vi "MysqlTest2 (2).vi"() -> ()   [LabVIEW 2018]
uses:
  Subvi/TheConnWithOmron/Panel_IO.ctl
  Subvi/TheConnWithOmron/Panel_IO2.ctl
  <vilib>/addons/database/Connection.llb/DB Tools Open Connec (String).vi
  <vilib>/addons/database/NI_Database_API.lvlib
panel:
  out "连接的字符串":string
  in  "终止":bool
  in  "左侧菜单选项卡":T1
  in  "重新连接":bool
  out "连接信号":bool
  in  "用户变更":bool
  in  "请选择用户:":enum16{"", "Operator", "Administrator"}(ring)
  in  "请输入密码:":string
  in  "确认变更":bool
  out "当前用户:":enum16{"Null", "Operator", "Administrator"}(ring)
  in  "用户登出":bool
  out "伺服参数监控":string[](array[string])
  in  "4":bool
  in  "3":bool
  in  "2":bool
  in  "1":bool
  in  "主界面选项卡":enum32{"IO监控", "参数设置", "手动操作", "数据管理", "调试界面"}(tab)
  in  "IO监控滚动条":i32(c297)
  out "Input":T2
  out "Output":T3
  in  "查询":bool
  in  "终结时间":timestamp
  in  "起始时间":timestamp
  in  "关键字查询":string
  in  "刷新":bool
  out "当前页数":i16
  out "总页数":i16
  in  "下一页":bool
  in  "上一页":bool
  out "数据查询":string[][](table)
  out "data":string[][](table)
  out "error out":errorcluster caption="错误输出"
  out "ExcelOutputData":string[](array[string])
  out "ExcelInputData":string[](array[string])
  out "InputData":string[][](array[string])
  out "引用输出":refnum<k24>
  out "OuputData":string[][](array[string])
  out "MachineCondition":string[][](array[string])
  # "mm"
  # "X1Pos:"
  # "mm"
  # "X2Pos:"
  # "mm"
  # "X3Pos:"
  # "mm"
  # "X4Pos:"
  # "mm"
  # "X5Pos:"
  # "mm"
  # "X6Pos:"
  # "mm"
  # "X7Pos:"
  # "mm/s"
  # "X1Vel:"
  # "mm/s"
  # "X2Vel:"
  # "mm/s"
  # "X3Vel:"
  # "mm/s"
  # "X4Vel:"
  # "mm/s"
  # "X5Vel:"
  # "mm/s"
  # "X6Vel:"
  # "mm/s"
  # "X7Vel:"
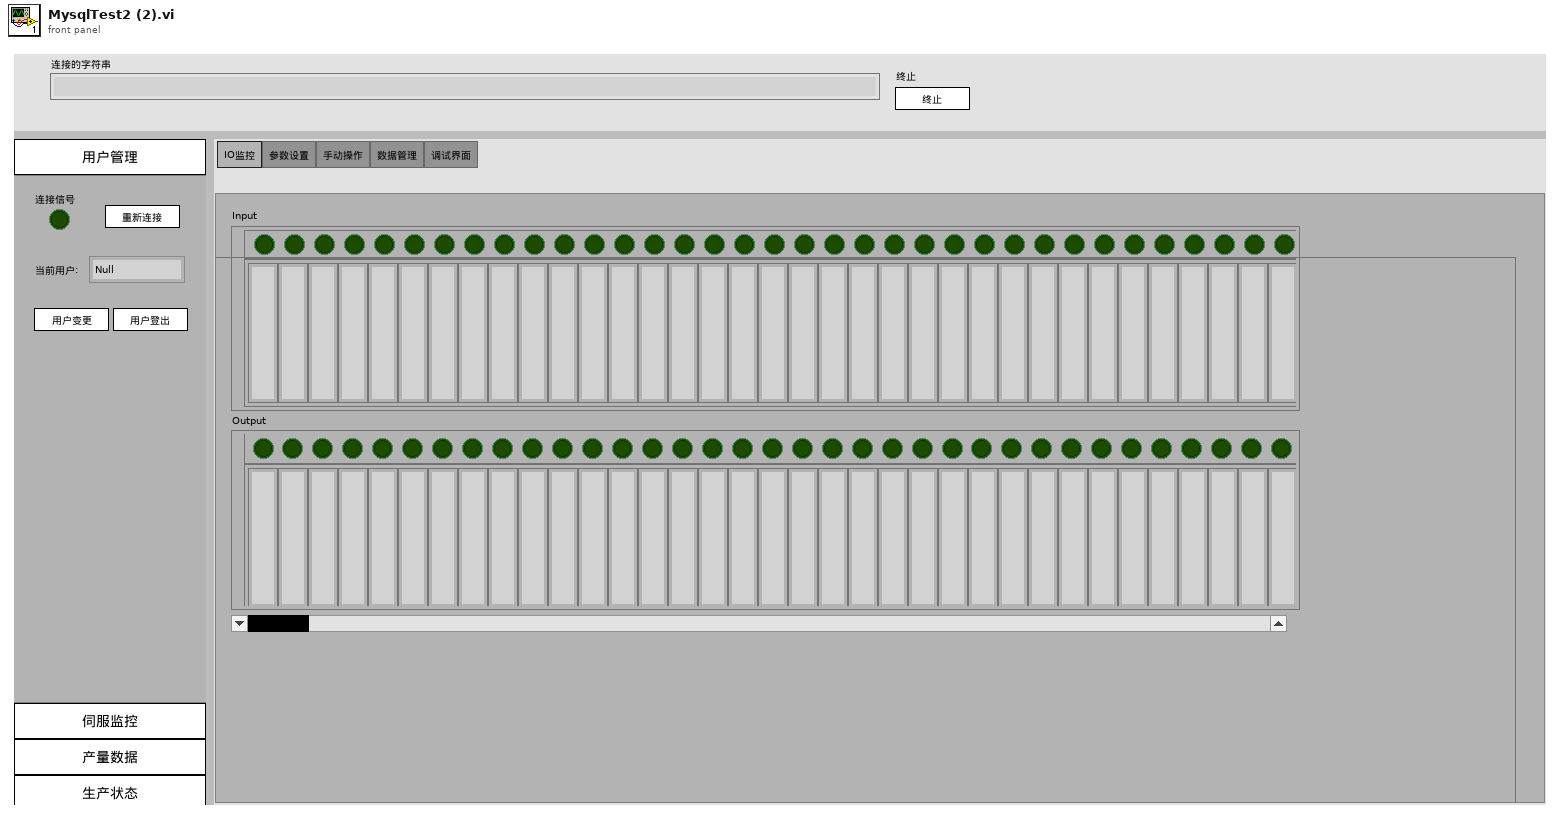
[diagram p1: front panel]
types:
  T1 = typedef "左侧菜单栏选项卡.ctl" = enum32{"用户管理", "伺服监控", "产量数据", "状态监控"}
  T2 = typedef "Panel_IO2.ctl" = cluster{"InputContent":cluster{"InputContent[0]":bool, "InputContent[1]":bool, "InputContent[2]":bool, "InputContent[3]":bool, "InputContent[4]":bool, "InputContent[5]":bool, "InputContent[6]":bool, "InputContent[7]":bool, "InputContent[8]":bool, "InputContent[9]":bool, "InputContent[10]":bool, "InputContent[11]":bool, "InputContent[12]":bool, "InputContent[13]":bool, "InputContent[14]":bool, "InputContent[15]":bool, "InputContent[16]":bool, "InputContent[17]":bool, "InputContent[18]":bool, "InputContent[19]":bool, "InputContent[20]":bool, "InputContent[21]":bool, "InputContent[22]":bool, "InputContent[23]":bool, "InputContent[24]":bool, "InputContent[25]":bool, "InputContent[26]":bool, "InputContent[27]":bool, "InputContent[28]":bool, "InputContent[29]":bool, "InputContent[30]":bool, "InputContent[31]":bool, "InputContent[32]":bool, "InputContent[33]":bool, "InputContent[34]":bool, "InputContent[35]":bool, "InputContent[36]":bool, "InputContent[37]":bool, "InputContent[38]":bool, "InputContent[39]":bool, "InputContent[40]":bool, "InputContent[41]":bool, "InputContent[42]":bool, "InputContent[43]":bool, "InputContent[44]":bool, "InputContent[45]":bool, "InputContent[46]":bool, "InputContent[47]":bool, "InputContent[48]":bool, "InputContent[49]":bool, "InputContent[50]":bool, "InputContent[51]":bool, "InputContent[52]":bool, "InputContent[53]":bool, "InputContent[54]":bool, "InputContent[55]":bool, "InputContent[56]":bool, "InputContent[57]":bool, "InputContent[58]":bool, "InputContent[59]":bool, "InputContent[60]":bool, "InputContent[61]":bool, "InputContent[62]":bool, "InputContent[63]":bool, "InputContent[64]":bool, "InputContent[65]":bool, "InputContent[66]":bool, "InputContent[67]":bool, "InputContent[68]":bool, "InputContent[69]":bool, "InputContent[70]":bool, "InputContent[71]":bool}, "ExcelInputData":cluster{"ExcelInputData[0]":string, "ExcelInputData[1]":string, "ExcelInputData[2]":string, "ExcelInputData[3]":string, "ExcelInputData[4]":string, "ExcelInputData[5]":string, "ExcelInputData[6]":string, "ExcelInputData[7]":string, "ExcelInputData[8]":string, "ExcelInputData[9]":string, "ExcelInputData[10]":string, "ExcelInputData[11]":string, "ExcelInputData[12]":string, "ExcelInputData[13]":string, "ExcelInputData[14]":string, "ExcelInputData[15]":string, "ExcelInputData[16]":string, "ExcelInputData[17]":string, "ExcelInputData[18]":string, "ExcelInputData[19]":string, "ExcelInputData[20]":string, "ExcelInputData[21]":string, "ExcelInputData[22]":string, "ExcelInputData[23]":string, "ExcelInputData[24]":string, "ExcelInputData[25]":string, "ExcelInputData[26]":string, "ExcelInputData[27]":string, "ExcelInputData[28]":string, "ExcelInputData[29]":string, "ExcelInputData[30]":string, "ExcelInputData[31]":string, "ExcelInputData[32]":string, "ExcelInputData[33]":string, "ExcelInputData[34]":string, "ExcelInputData[35]":string, "ExcelInputData[36]":string, "ExcelInputData[37]":string, "ExcelInputData[38]":string, "ExcelInputData[39]":string, "ExcelInputData[40]":string, "ExcelInputData[41]":string, "ExcelInputData[42]":string, "ExcelInputData[43]":string, "ExcelInputData[44]":string, "ExcelInputData[45]":string, "ExcelInputData[46]":string, "ExcelInputData[47]":string, "ExcelInputData[48]":string, "ExcelInputData[49]":string, "ExcelInputData[50]":string, "ExcelInputData[51]":string, "ExcelInputData[52]":string, "ExcelInputData[53]":string, "ExcelInputData[54]":string, "ExcelInputData[55]":string, "ExcelInputData[56]":string, "ExcelInputData[57]":string, "ExcelInputData[58]":string, "ExcelInputData[59]":string, "ExcelInputData[60]":string, "ExcelInputData[61]":string, "ExcelInputData[62]":string, "ExcelInputData[63]":string, "ExcelInputData[64]":string, "ExcelInputData[65]":string, "ExcelInputData[66]":string, "ExcelInputData[67]":string, "ExcelInputData[68]":string, "ExcelInputData[69]":string, "ExcelInputData[70]":string, "ExcelInputData[71]":string}}
  T3 = typedef "Panel_IO.ctl" = cluster{"OutputContent":cluster{"OutputContent[0]":bool, "OutputContent[1]":bool, "OutputContent[2]":bool, "OutputContent[3]":bool, "OutputContent[4]":bool, "OutputContent[5]":bool, "OutputContent[6]":bool, "OutputContent[7]":bool, "OutputContent[8]":bool, "OutputContent[9]":bool, "OutputContent[10]":bool, "OutputContent[11]":bool, "OutputContent[12]":bool, "OutputContent[13]":bool, "OutputContent[14]":bool, "OutputContent[15]":bool, "OutputContent[16]":bool, "OutputContent[17]":bool, "OutputContent[18]":bool, "OutputContent[19]":bool, "OutputContent[20]":bool, "OutputContent[21]":bool, "OutputContent[22]":bool, "OutputContent[23]":bool, "OutputContent[24]":bool, "OutputContent[25]":bool, "OutputContent[26]":bool, "OutputContent[27]":bool, "OutputContent[28]":bool, "OutputContent[29]":bool, "OutputContent[30]":bool, "OutputContent[31]":bool, "OutputContent[32]":bool, "OutputContent[33]":bool, "OutputContent[34]":bool, "OutputContent[35]":bool, "OutputContent[36]":bool, "OutputContent[37]":bool, "OutputContent[38]":bool, "OutputContent[39]":bool, "OutputContent[40]":bool, "OutputContent[41]":bool, "OutputContent[42]":bool, "OutputContent[43]":bool, "OutputContent[44]":bool, "OutputContent[45]":bool, "OutputContent[46]":bool, "OutputContent[47]":bool}, "ExcelOutputData":cluster{"ExcelOutputData[0]":string, "ExcelOutputData[1]":string, "ExcelOutputData[2]":string, "ExcelOutputData[3]":string, "ExcelOutputData[4]":string, "ExcelOutputData[5]":string, "ExcelOutputData[6]":string, "ExcelOutputData[7]":string, "ExcelOutputData[8]":string, "ExcelOutputData[9]":string, "ExcelOutputData[10]":string, "ExcelOutputData[11]":string, "ExcelOutputData[12]":string, "ExcelOutputData[13]":string, "ExcelOutputData[14]":string, "ExcelOutputData[15]":string, "ExcelOutputData[16]":string, "ExcelOutputData[17]":string, "ExcelOutputData[18]":string, "ExcelOutputData[19]":string, "ExcelOutputData[20]":string, "ExcelOutputData[21]":string, "ExcelOutputData[22]":string, "ExcelOutputData[23]":string, "ExcelOutputData[24]":string, "ExcelOutputData[25]":string, "ExcelOutputData[26]":string, "ExcelOutputData[27]":string, "ExcelOutputData[28]":string, "ExcelOutputData[29]":string, "ExcelOutputData[30]":string, "ExcelOutputData[31]":string, "ExcelOutputData[32]":string, "ExcelOutputData[33]":string, "ExcelOutputData[34]":string, "ExcelOutputData[35]":string, "ExcelOutputData[36]":string, "ExcelOutputData[37]":string, "ExcelOutputData[38]":string, "ExcelOutputData[39]":string, "ExcelOutputData[40]":string, "ExcelOutputData[41]":string, "ExcelOutputData[42]":string, "ExcelOutputData[43]":string, "ExcelOutputData[44]":string, "ExcelOutputData[45]":string, "ExcelOutputData[46]":string, "ExcelOutputData[47]":string}}
  T4 = typedef "imagedata.ctl" = cluster{"image type":i32, "image depth":i32, "image":u8[], "mask":u8[], "colors":u32[], "Rectangle":cluster{"left":i16, "top":i16, "right":i16, "bottom":i16}}
  T5 = enum16{"inti", "NormalWork", "errorConnect?", "inti_excel"}
  T6 = cluster{"InputContent[0]":bool, "InputContent[1]":bool, "InputContent[2]":bool, "InputContent[3]":bool, "InputContent[4]":bool, "InputContent[5]":bool, "InputContent[6]":bool, "InputContent[7]":bool, "InputContent[8]":bool, "InputContent[9]":bool, "InputContent[10]":bool, "InputContent[11]":bool, "InputContent[12]":bool, "InputContent[13]":bool, "InputContent[14]":bool, "InputContent[15]":bool, "InputContent[16]":bool, "InputContent[17]":bool, "InputContent[18]":bool, "InputContent[19]":bool, "InputContent[20]":bool, "InputContent[21]":bool, "InputContent[22]":bool, "InputContent[23]":bool, "InputContent[24]":bool, "InputContent[25]":bool, "InputContent[26]":bool, "InputContent[27]":bool, "InputContent[28]":bool, "InputContent[29]":bool, "InputContent[30]":bool, "InputContent[31]":bool, "InputContent[32]":bool, "InputContent[33]":bool, "InputContent[34]":bool, "InputContent[35]":bool, "InputContent[36]":bool, "InputContent[37]":bool, "InputContent[38]":bool, "InputContent[39]":bool, "InputContent[40]":bool, "InputContent[41]":bool, "InputContent[42]":bool, "InputContent[43]":bool, "InputContent[44]":bool, "InputContent[45]":bool, "InputContent[46]":bool, "InputContent[47]":bool, "InputContent[48]":bool, "InputContent[49]":bool, "InputContent[50]":bool, "InputContent[51]":bool, "InputContent[52]":bool, "InputContent[53]":bool, "InputContent[54]":bool, "InputContent[55]":bool, "InputContent[56]":bool, "InputContent[57]":bool, "InputContent[58]":bool, "InputContent[59]":bool, "InputContent[60]":bool, "InputContent[61]":bool, "InputContent[62]":bool, "InputContent[63]":bool, "InputContent[64]":bool, "InputContent[65]":bool, "InputContent[66]":bool, "InputContent[67]":bool, "InputContent[68]":bool, "InputContent[69]":bool, "InputContent[70]":bool, "InputContent[71]":bool}
  T7 = cluster{"ExcelInputData[0]":string, "ExcelInputData[1]":string, "ExcelInputData[2]":string, "ExcelInputData[3]":string, "ExcelInputData[4]":string, "ExcelInputData[5]":string, "ExcelInputData[6]":string, "ExcelInputData[7]":string, "ExcelInputData[8]":string, "ExcelInputData[9]":string, "ExcelInputData[10]":string, "ExcelInputData[11]":string, "ExcelInputData[12]":string, "ExcelInputData[13]":string, "ExcelInputData[14]":string, "ExcelInputData[15]":string, "ExcelInputData[16]":string, "ExcelInputData[17]":string, "ExcelInputData[18]":string, "ExcelInputData[19]":string, "ExcelInputData[20]":string, "ExcelInputData[21]":string, "ExcelInputData[22]":string, "ExcelInputData[23]":string, "ExcelInputData[24]":string, "ExcelInputData[25]":string, "ExcelInputData[26]":string, "ExcelInputData[27]":string, "ExcelInputData[28]":string, "ExcelInputData[29]":string, "ExcelInputData[30]":string, "ExcelInputData[31]":string, "ExcelInputData[32]":string, "ExcelInputData[33]":string, "ExcelInputData[34]":string, "ExcelInputData[35]":string, "ExcelInputData[36]":string, "ExcelInputData[37]":string, "ExcelInputData[38]":string, "ExcelInputData[39]":string, "ExcelInputData[40]":string, "ExcelInputData[41]":string, "ExcelInputData[42]":string, "ExcelInputData[43]":string, "ExcelInputData[44]":string, "ExcelInputData[45]":string, "ExcelInputData[46]":string, "ExcelInputData[47]":string, "ExcelInputData[48]":string, "ExcelInputData[49]":string, "ExcelInputData[50]":string, "ExcelInputData[51]":string, "ExcelInputData[52]":string, "ExcelInputData[53]":string, "ExcelInputData[54]":string, "ExcelInputData[55]":string, "ExcelInputData[56]":string, "ExcelInputData[57]":string, "ExcelInputData[58]":string, "ExcelInputData[59]":string, "ExcelInputData[60]":string, "ExcelInputData[61]":string, "ExcelInputData[62]":string, "ExcelInputData[63]":string, "ExcelInputData[64]":string, "ExcelInputData[65]":string, "ExcelInputData[66]":string, "ExcelInputData[67]":string, "ExcelInputData[68]":string, "ExcelInputData[69]":string, "ExcelInputData[70]":string, "ExcelInputData[71]":string}
  T8 = cluster{"OutputContent[0]":bool, "OutputContent[1]":bool, "OutputContent[2]":bool, "OutputContent[3]":bool, "OutputContent[4]":bool, "OutputContent[5]":bool, "OutputContent[6]":bool, "OutputContent[7]":bool, "OutputContent[8]":bool, "OutputContent[9]":bool, "OutputContent[10]":bool, "OutputContent[11]":bool, "OutputContent[12]":bool, "OutputContent[13]":bool, "OutputContent[14]":bool, "OutputContent[15]":bool, "OutputContent[16]":bool, "OutputContent[17]":bool, "OutputContent[18]":bool, "OutputContent[19]":bool, "OutputContent[20]":bool, "OutputContent[21]":bool, "OutputContent[22]":bool, "OutputContent[23]":bool, "OutputContent[24]":bool, "OutputContent[25]":bool, "OutputContent[26]":bool, "OutputContent[27]":bool, "OutputContent[28]":bool, "OutputContent[29]":bool, "OutputContent[30]":bool, "OutputContent[31]":bool, "OutputContent[32]":bool, "OutputContent[33]":bool, "OutputContent[34]":bool, "OutputContent[35]":bool, "OutputContent[36]":bool, "OutputContent[37]":bool, "OutputContent[38]":bool, "OutputContent[39]":bool, "OutputContent[40]":bool, "OutputContent[41]":bool, "OutputContent[42]":bool, "OutputContent[43]":bool, "OutputContent[44]":bool, "OutputContent[45]":bool, "OutputContent[46]":bool, "OutputContent[47]":bool}
  T9 = cluster{"ExcelOutputData[0]":string, "ExcelOutputData[1]":string, "ExcelOutputData[2]":string, "ExcelOutputData[3]":string, "ExcelOutputData[4]":string, "ExcelOutputData[5]":string, "ExcelOutputData[6]":string, "ExcelOutputData[7]":string, "ExcelOutputData[8]":string, "ExcelOutputData[9]":string, "ExcelOutputData[10]":string, "ExcelOutputData[11]":string, "ExcelOutputData[12]":string, "ExcelOutputData[13]":string, "ExcelOutputData[14]":string, "ExcelOutputData[15]":string, "ExcelOutputData[16]":string, "ExcelOutputData[17]":string, "ExcelOutputData[18]":string, "ExcelOutputData[19]":string, "ExcelOutputData[20]":string, "ExcelOutputData[21]":string, "ExcelOutputData[22]":string, "ExcelOutputData[23]":string, "ExcelOutputData[24]":string, "ExcelOutputData[25]":string, "ExcelOutputData[26]":string, "ExcelOutputData[27]":string, "ExcelOutputData[28]":string, "ExcelOutputData[29]":string, "ExcelOutputData[30]":string, "ExcelOutputData[31]":string, "ExcelOutputData[32]":string, "ExcelOutputData[33]":string, "ExcelOutputData[34]":string, "ExcelOutputData[35]":string, "ExcelOutputData[36]":string, "ExcelOutputData[37]":string, "ExcelOutputData[38]":string, "ExcelOutputData[39]":string, "ExcelOutputData[40]":string, "ExcelOutputData[41]":string, "ExcelOutputData[42]":string, "ExcelOutputData[43]":string, "ExcelOutputData[44]":string, "ExcelOutputData[45]":string, "ExcelOutputData[46]":string, "ExcelOutputData[47]":string}
  T10 = cluster{"InputContent":cluster{"InputContent[0]":bool, "InputContent[1]":bool, "InputContent[2]":bool, "InputContent[3]":bool, "InputContent[4]":bool, "InputContent[5]":bool, "InputContent[6]":bool, "InputContent[7]":bool, "InputContent[8]":bool, "InputContent[9]":bool, "InputContent[10]":bool, "InputContent[11]":bool, "InputContent[12]":bool, "InputContent[13]":bool, "InputContent[14]":bool, "InputContent[15]":bool, "InputContent[16]":bool, "InputContent[17]":bool, "InputContent[18]":bool, "InputContent[19]":bool, "InputContent[20]":bool, "InputContent[21]":bool, "InputContent[22]":bool, "InputContent[23]":bool, "InputContent[24]":bool, "InputContent[25]":bool, "InputContent[26]":bool, "InputContent[27]":bool, "InputContent[28]":bool, "InputContent[29]":bool, "InputContent[30]":bool, "InputContent[31]":bool, "InputContent[32]":bool, "InputContent[33]":bool, "InputContent[34]":bool, "InputContent[35]":bool, "InputContent[36]":bool, "InputContent[37]":bool, "InputContent[38]":bool, "InputContent[39]":bool, "InputContent[40]":bool, "InputContent[41]":bool, "InputContent[42]":bool, "InputContent[43]":bool, "InputContent[44]":bool, "InputContent[45]":bool, "InputContent[46]":bool, "InputContent[47]":bool, "InputContent[48]":bool, "InputContent[49]":bool, "InputContent[50]":bool, "InputContent[51]":bool, "InputContent[52]":bool, "InputContent[53]":bool, "InputContent[54]":bool, "InputContent[55]":bool, "InputContent[56]":bool, "InputContent[57]":bool, "InputContent[58]":bool, "InputContent[59]":bool, "InputContent[60]":bool, "InputContent[61]":bool, "InputContent[62]":bool, "InputContent[63]":bool, "InputContent[64]":bool, "InputContent[65]":bool, "InputContent[66]":bool, "InputContent[67]":bool, "InputContent[68]":bool, "InputContent[69]":bool, "InputContent[70]":bool, "InputContent[71]":bool}, "ExcelInputData":cluster{"ExcelInputData[0]":string, "ExcelInputData[1]":string, "ExcelInputData[2]":string, "ExcelInputData[3]":string, "ExcelInputData[4]":string, "ExcelInputData[5]":string, "ExcelInputData[6]":string, "ExcelInputData[7]":string, "ExcelInputData[8]":string, "ExcelInputData[9]":string, "ExcelInputData[10]":string, "ExcelInputData[11]":string, "ExcelInputData[12]":string, "ExcelInputData[13]":string, "ExcelInputData[14]":string, "ExcelInputData[15]":string, "ExcelInputData[16]":string, "ExcelInputData[17]":string, "ExcelInputData[18]":string, "ExcelInputData[19]":string, "ExcelInputData[20]":string, "ExcelInputData[21]":string, "ExcelInputData[22]":string, "ExcelInputData[23]":string, "ExcelInputData[24]":string, "ExcelInputData[25]":string, "ExcelInputData[26]":string, "ExcelInputData[27]":string, "ExcelInputData[28]":string, "ExcelInputData[29]":string, "ExcelInputData[30]":string, "ExcelInputData[31]":string, "ExcelInputData[32]":string, "ExcelInputData[33]":string, "ExcelInputData[34]":string, "ExcelInputData[35]":string, "ExcelInputData[36]":string, "ExcelInputData[37]":string, "ExcelInputData[38]":string, "ExcelInputData[39]":string, "ExcelInputData[40]":string, "ExcelInputData[41]":string, "ExcelInputData[42]":string, "ExcelInputData[43]":string, "ExcelInputData[44]":string, "ExcelInputData[45]":string, "ExcelInputData[46]":string, "ExcelInputData[47]":string, "ExcelInputData[48]":string, "ExcelInputData[49]":string, "ExcelInputData[50]":string, "ExcelInputData[51]":string, "ExcelInputData[52]":string, "ExcelInputData[53]":string, "ExcelInputData[54]":string, "ExcelInputData[55]":string, "ExcelInputData[56]":string, "ExcelInputData[57]":string, "ExcelInputData[58]":string, "ExcelInputData[59]":string, "ExcelInputData[60]":string, "ExcelInputData[61]":string, "ExcelInputData[62]":string, "ExcelInputData[63]":string, "ExcelInputData[64]":string, "ExcelInputData[65]":string, "ExcelInputData[66]":string, "ExcelInputData[67]":string, "ExcelInputData[68]":string, "ExcelInputData[69]":string, "ExcelInputData[70]":string, "ExcelInputData[71]":string}}
  T11 = cluster{"OutputContent":cluster{"OutputContent[0]":bool, "OutputContent[1]":bool, "OutputContent[2]":bool, "OutputContent[3]":bool, "OutputContent[4]":bool, "OutputContent[5]":bool, "OutputContent[6]":bool, "OutputContent[7]":bool, "OutputContent[8]":bool, "OutputContent[9]":bool, "OutputContent[10]":bool, "OutputContent[11]":bool, "OutputContent[12]":bool, "OutputContent[13]":bool, "OutputContent[14]":bool, "OutputContent[15]":bool, "OutputContent[16]":bool, "OutputContent[17]":bool, "OutputContent[18]":bool, "OutputContent[19]":bool, "OutputContent[20]":bool, "OutputContent[21]":bool, "OutputContent[22]":bool, "OutputContent[23]":bool, "OutputContent[24]":bool, "OutputContent[25]":bool, "OutputContent[26]":bool, "OutputContent[27]":bool, "OutputContent[28]":bool, "OutputContent[29]":bool, "OutputContent[30]":bool, "OutputContent[31]":bool, "OutputContent[32]":bool, "OutputContent[33]":bool, "OutputContent[34]":bool, "OutputContent[35]":bool, "OutputContent[36]":bool, "OutputContent[37]":bool, "OutputContent[38]":bool, "OutputContent[39]":bool, "OutputContent[40]":bool, "OutputContent[41]":bool, "OutputContent[42]":bool, "OutputContent[43]":bool, "OutputContent[44]":bool, "OutputContent[45]":bool, "OutputContent[46]":bool, "OutputContent[47]":bool}, "ExcelOutputData":cluster{"ExcelOutputData[0]":string, "ExcelOutputData[1]":string, "ExcelOutputData[2]":string, "ExcelOutputData[3]":string, "ExcelOutputData[4]":string, "ExcelOutputData[5]":string, "ExcelOutputData[6]":string, "ExcelOutputData[7]":string, "ExcelOutputData[8]":string, "ExcelOutputData[9]":string, "ExcelOutputData[10]":string, "ExcelOutputData[11]":string, "ExcelOutputData[12]":string, "ExcelOutputData[13]":string, "ExcelOutputData[14]":string, "ExcelOutputData[15]":string, "ExcelOutputData[16]":string, "ExcelOutputData[17]":string, "ExcelOutputData[18]":string, "ExcelOutputData[19]":string, "ExcelOutputData[20]":string, "ExcelOutputData[21]":string, "ExcelOutputData[22]":string, "ExcelOutputData[23]":string, "ExcelOutputData[24]":string, "ExcelOutputData[25]":string, "ExcelOutputData[26]":string, "ExcelOutputData[27]":string, "ExcelOutputData[28]":string, "ExcelOutputData[29]":string, "ExcelOutputData[30]":string, "ExcelOutputData[31]":string, "ExcelOutputData[32]":string, "ExcelOutputData[33]":string, "ExcelOutputData[34]":string, "ExcelOutputData[35]":string, "ExcelOutputData[36]":string, "ExcelOutputData[37]":string, "ExcelOutputData[38]":string, "ExcelOutputData[39]":string, "ExcelOutputData[40]":string, "ExcelOutputData[41]":string, "ExcelOutputData[42]":string, "ExcelOutputData[43]":string, "ExcelOutputData[44]":string, "ExcelOutputData[45]":string, "ExcelOutputData[46]":string, "ExcelOutputData[47]":string}}
  T12 = typedef "NI_Database_API.lvlib/Conn ObjectReference.ctl" = refnum<k1>
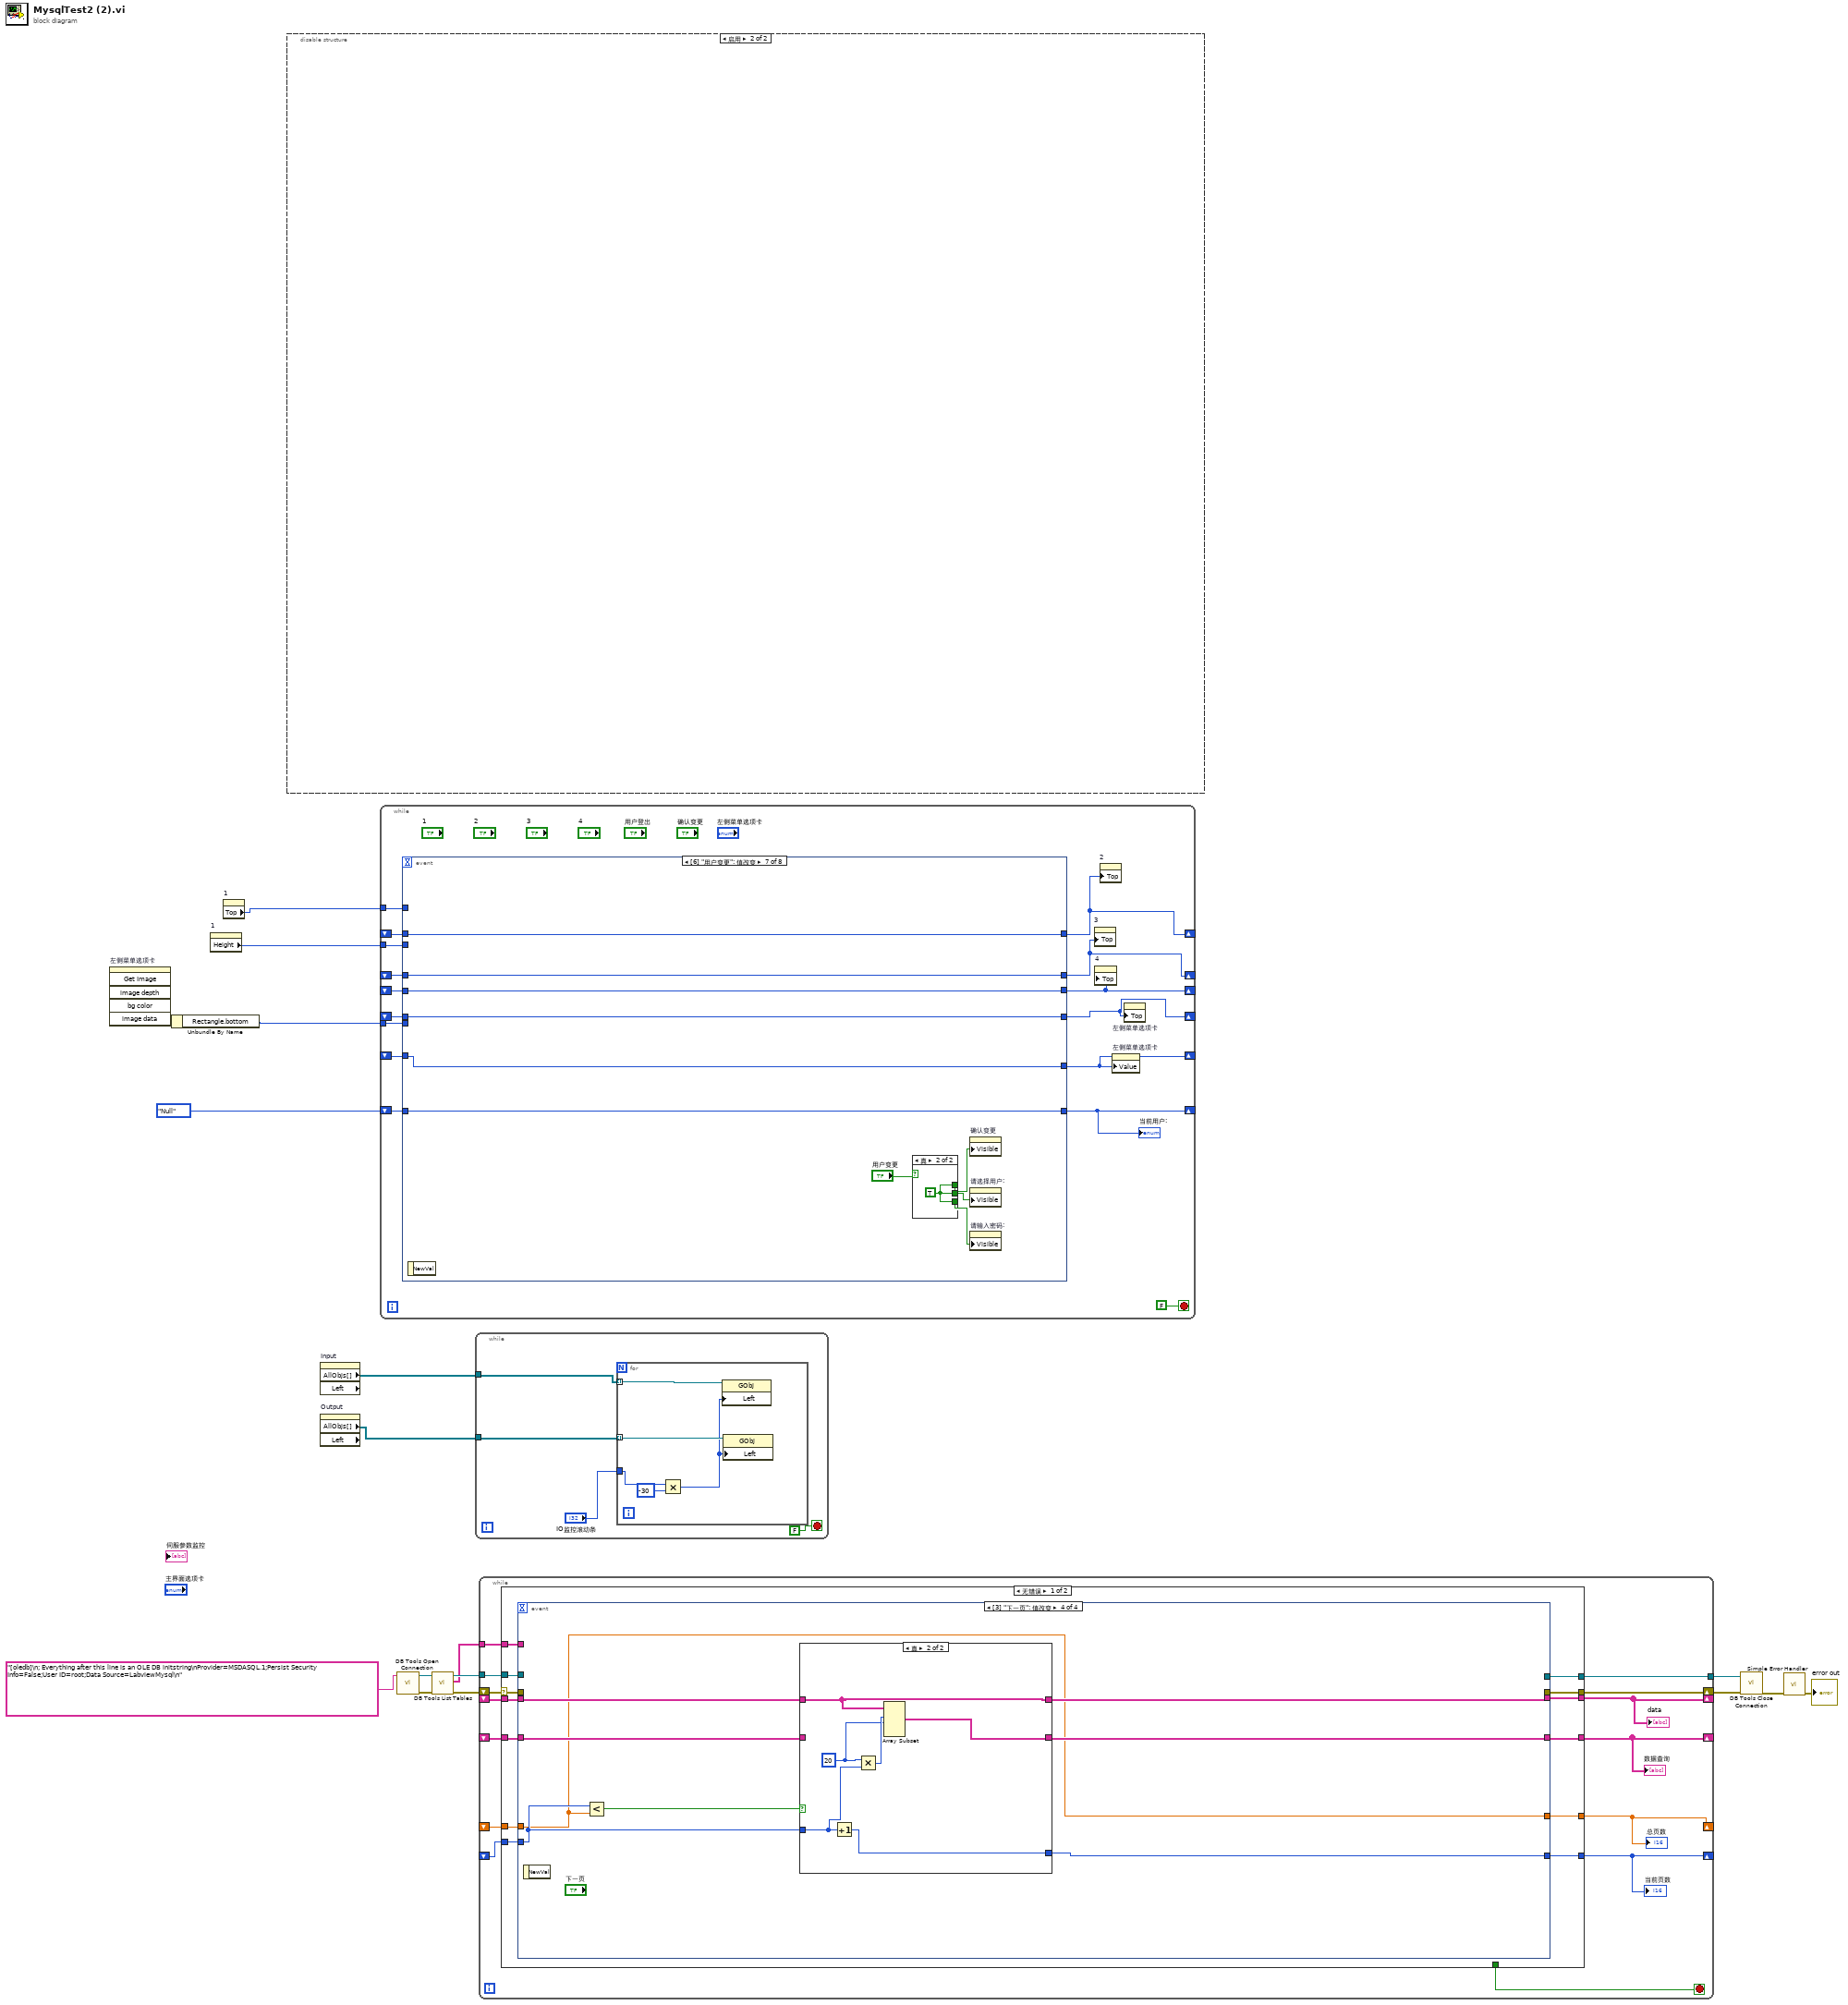
[diagram p0: block diagram]
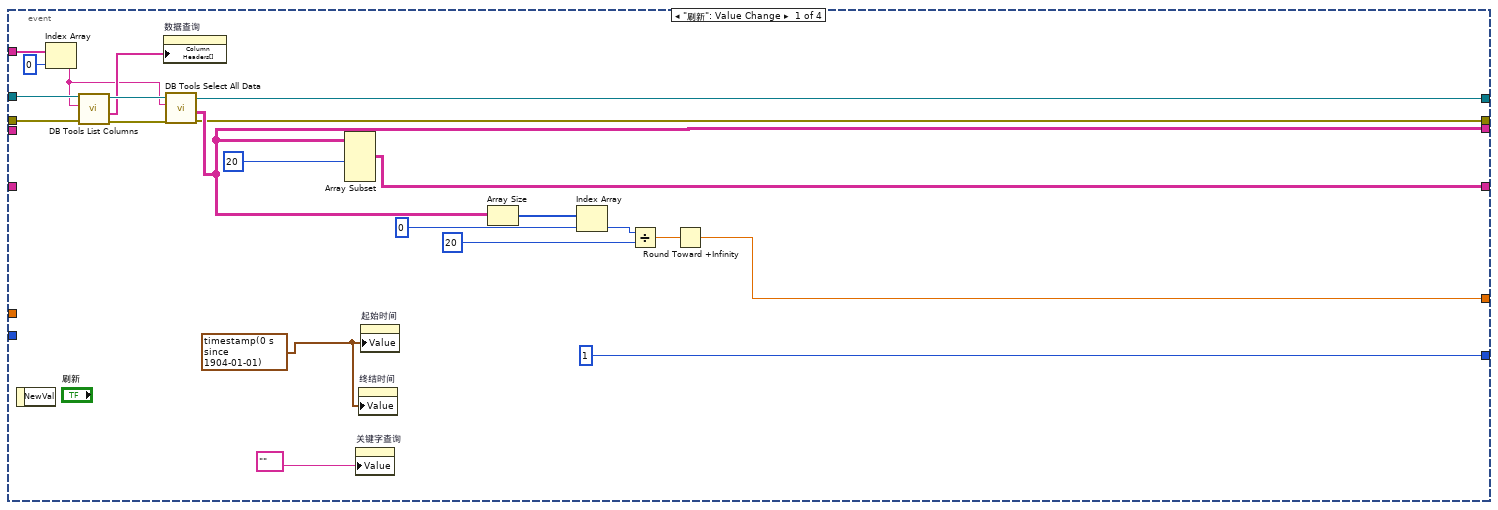
[diagram p2: hidden frame]
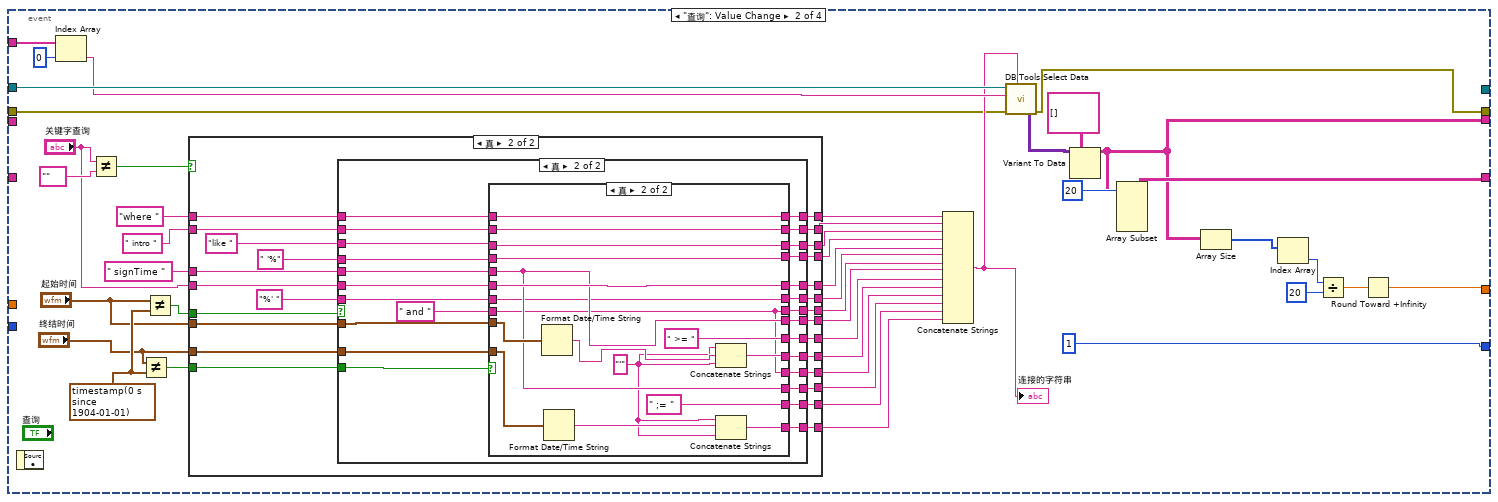
[diagram p3: hidden frame]
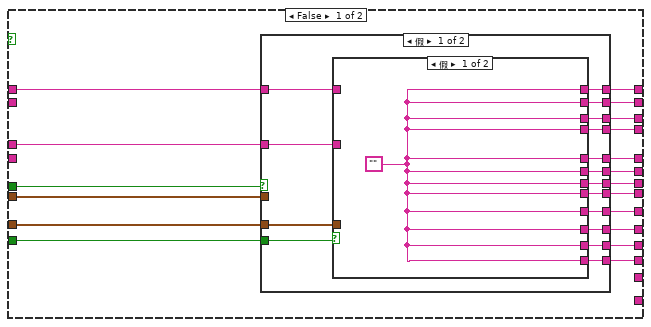
[diagram p4: hidden frame]
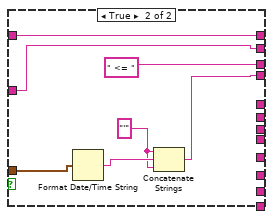
[diagram p5: hidden frame]
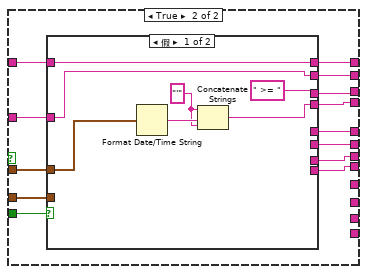
[diagram p6: hidden frame]
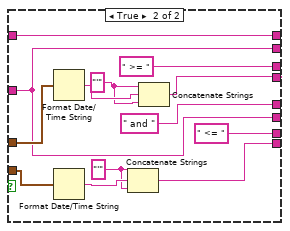
[diagram p7: hidden frame]
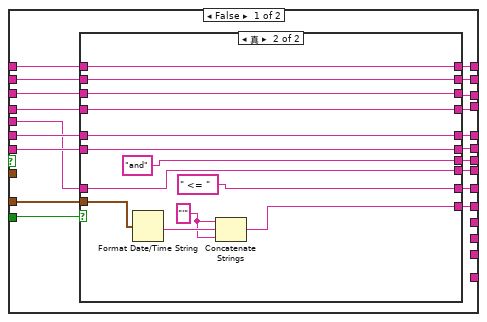
[diagram p8: hidden frame]
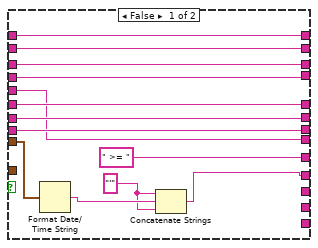
[diagram p10: hidden frame]
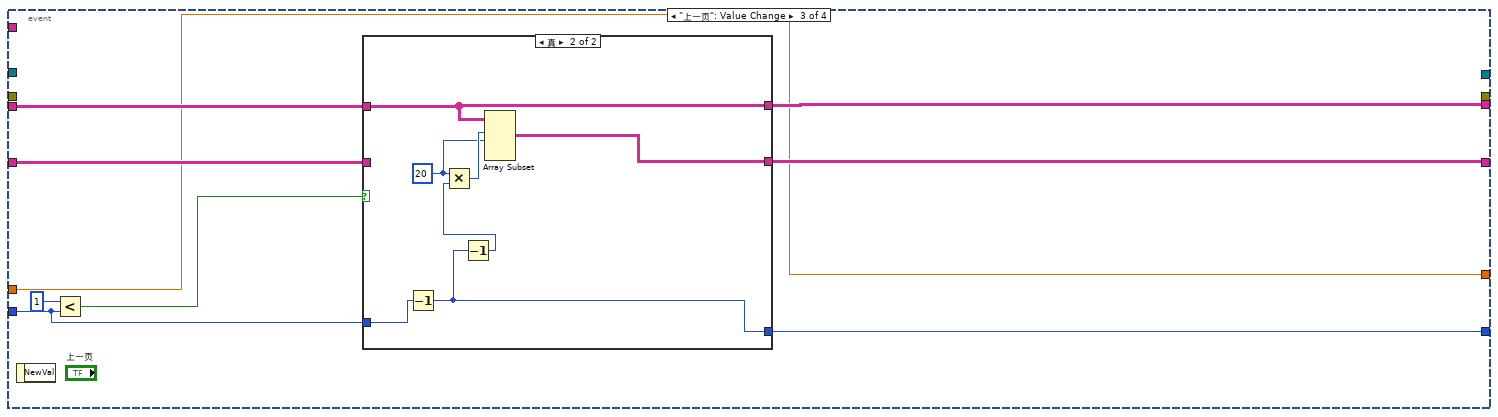
[diagram p11: hidden frame]
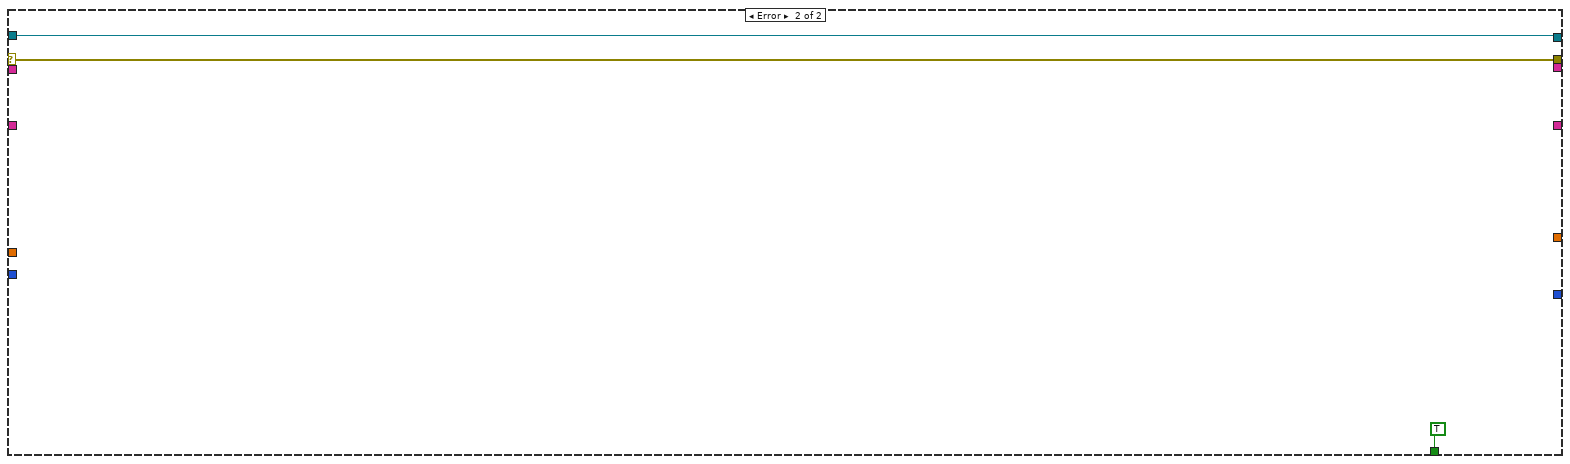
[diagram p14: hidden frame]
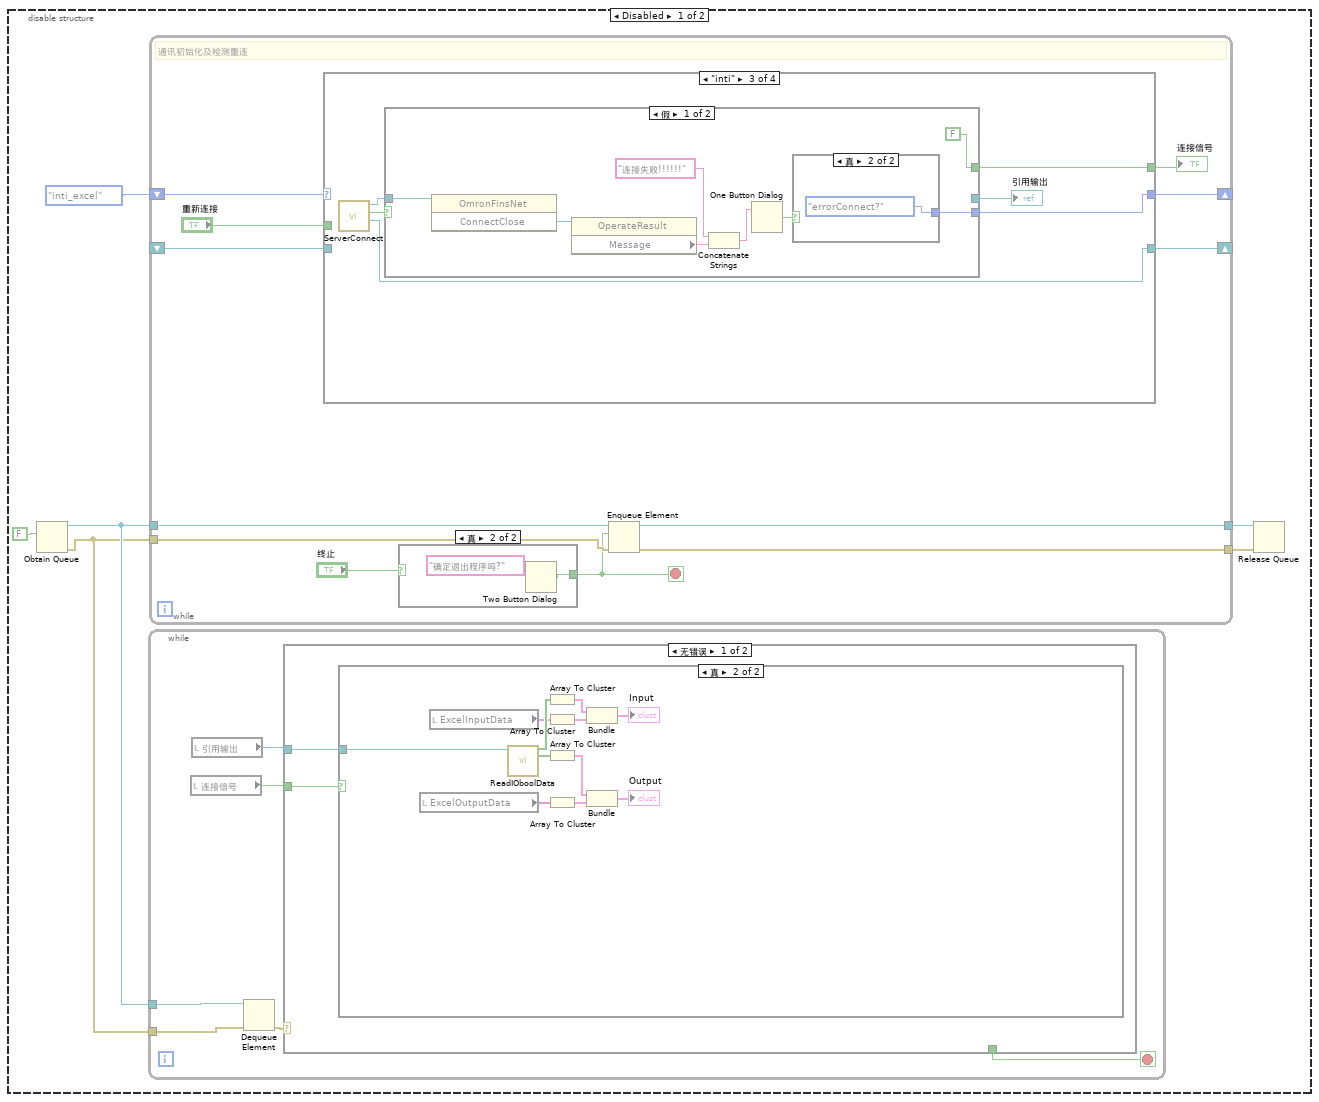
[diagram p15: hidden frame]
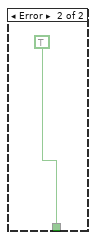
[diagram p17: hidden frame]
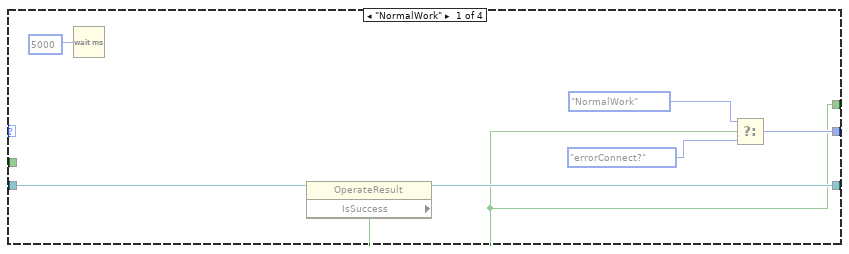
[diagram p19: hidden frame]
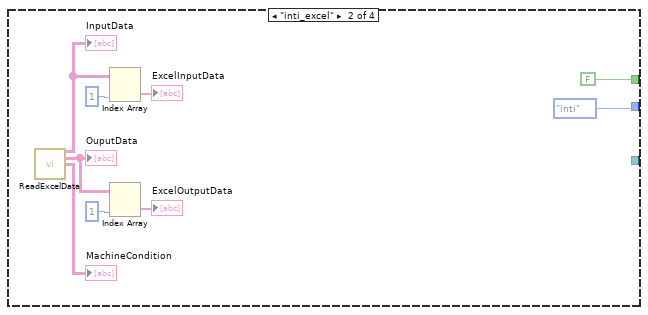
[diagram p20: hidden frame]
diagram:
  n1 = invoke on="左侧菜单选项卡" class="TabCtl (严格)" method="Get Image"() -> ("image data"=w15:T4)  [unwired: 6 in, 5 out]
  n2 = Unbundle By Name(w15) -> ("Rectangle.bottom"=w14:i16)
  n3 = property on="1" class="Bool"() -> ("Height"=w16:u32)  [unwired: 2 in, 2 out]
  n4 = property on="1" class="Bool"() -> ("Top"=w17:i32)  [unwired: 2 in, 2 out]
  n5 = disable-structure shown="启用" {
    frame Disabled {
      n6 = Obtain Queue(element data type=FALSE) -> (queue out=w19:refnum<queue>, error out=w18:errorcluster)  [unwired: 4 in, 1 out]
      n7 = while {
        tunnel: w18 -> [w27]
        tunnel: w19 -> [w28]
        stop <- w29 stop-if-true
        n8 = local read "连接信号"() -> (w25:bool)
        n9 = local read "引用输出"() -> (w24:refnum<k24>)
        n10 = Dequeue Element(queue=w28, error in (no error)=w27) -> (error out=w26:errorcluster)  [unwired: 1 in, 3 out]
        n11 = case shown="无错误" w26 {
          tunnel: [_ TRUE] -> w29
          tunnel: w24 -> [w31 _]
          tunnel: w25 -> [w30 _]
          frame No Error {
            n12 = case shown="真" w30 {
              tunnel: w31 -> [_ w42]
              frame False {
              }
              frame True {
                n13 = local read "ExcelOutputData"() -> (w39:string[])
                n14 = local read "ExcelInputData"() -> (w40:string[])
                n15 = call "ReadIOboolData.vi"("OmronFinsNet"=w42) -> ("InputContent"=w41:bool[], "OutputContent"=w38:bool[])  [unwired: 12 in, 1 out]
                n16 = Array To Cluster(array=w41) -> (cluster=w34:T6)
                n17 = Array To Cluster(array=w40) -> (cluster=w35:T7)
                n18 = Array To Cluster(array=w38) -> (cluster=w37:T8)
                n19 = Array To Cluster(array=w39) -> (cluster=w36:T9)
                n20 = Bundle("InputContent"=w34, "ExcelInputData"=w35) -> (→"Input":T10)  [unwired: 1 in]
                n21 = Bundle("OutputContent"=w37, "ExcelOutputData"=w36) -> (→"Output":T11)  [unwired: 1 in]
              }
            }
          }
          frame Error {
          }
        }
      }
      n22 = while {
        shift-right: [w55] -> _
        shift-left: T5."inti_excel" -> [w54]
        shift-right: [w52] -> _
        shift-left: _ -> [w51]
        tunnel: w19 -> [w50]
        tunnel: w18 -> [w49]
        tunnel: [w48] -> w21
        tunnel: [w47] -> w20
        stop <- w45 stop-if-true
        # "通讯初始化及检测重连"
        n23 = case shown="\"inti\"" w54 {
          tunnel: [w59 T5."inti" w76 w96] -> w55
          tunnel: [w58 FALSE w75 FALSE] -> w44
          tunnel: "重新连接" -> [_ _ _ w97]
          tunnel: [w62 _ w74 _] -> w52
          tunnel: w51 -> [w64 _ _ _]
          frame "NormalWork" {
            n24 = Wait (ms)(milliseconds to wait=u32 5000 ("等待时间（毫秒）")) -> ()  [unwired: 1 out]
            n25 = property class="OperateResult"(reference=w64) -> (reference out=w62:refnum<k24>, "IsSuccess"=w58:bool)  [unwired: 1 in, 1 out]
            n26 = Select(t=T5."NormalWork", s=w58, f=T5."errorConnect?") -> (s? t:f=w59:T5)
          }
          frame "inti_excel" {
            n27 = call "ReadExcelData.vi"() -> ("InputData"=w70:string[][], "OuputData"=w67:string[][], "MachineCondition"=→"MachineCondition":string[][])  [unwired: 12 in, 1 out]
            "InputData" <- w70
            "OuputData" <- w67
            n28 = Index Array(array=w70, index (col)=1 ("禁用的索引 (列)")) -> (element=→"ExcelInputData":string[])  [unwired: 1 in]
            n29 = Index Array(array=w67, index (col)=1 ("索引 (行)")) -> (element=→"ExcelOutputData":string[])  [unwired: 1 in]
          }
          frame "inti" {
            n30 = call "ServerConnect.vi"() -> ("ConnectServer"=w74:refnum<k24>, "IsSuccess"=w77:bool, "引用输出"=w78:refnum<k24>)  [unwired: 8 in, 1 out]
            n31 = case shown="假" w77 {
              tunnel: w78 -> [w85 w92]
              tunnel: [_ w92] -> w79
              tunnel: [w86 T5."NormalWork"] -> w76
              tunnel: [FALSE ("连接信号") TRUE ("连接信号")] -> w75
              frame False {
                n32 = invoke class="OmronFinsNet" method="ConnectClose"(reference=w85) -> ("ConnectClose"=w84:refnum<k24>)  [unwired: 2 in, 2 out]
                n33 = property class="OperateResult"(reference=w84) -> ("Message"=w83:string)  [unwired: 1 in, 2 out]
                n34 = Concatenate Strings("连接失败!!!!!!" ("消息"), w83) -> (w81:string)
                n35 = One Button Dialog(message=w81) -> (true=w87:bool)  [unwired: 1 in]
                n36 = case shown="真" w87 {
                  tunnel: [T5."errorConnect?" T5."errorConnect?"] -> w86
                  frame False {
                  }
                  frame True {
                  }
                }
              }
              frame True {
              }
            }
            "引用输出" <- w79
          }
          frame "errorConnect?", Default {
            n37 = Select(t=T5."inti", s=w97, f=T5."errorConnect?") -> (s? t:f=w96:T5)
          }
        }
        "连接信号" <- w44
        n38 = case shown="真" "终止" {
          tunnel: [_ w57] -> w45
          frame False {
          }
          frame True {
            n39 = Two Button Dialog(message="确定退出程序吗?" ("消息")) -> (T button?=w57:bool)  [unwired: 2 in]
          }
        }
        n40 = Enqueue Element(queue=w50, element=w45, error in (no error)=w49) -> (queue out=w48:refnum<queue>, error out=w47:errorcluster)  [unwired: 1 in, 1 out]
      }
      n41 = Release Queue(queue=w21, error in (no error)=w20) -> ()  [unwired: 1 in, 3 out]
    }
    frame Enabled {
    }
  }
  n42 = property on="Input" class="Clust (严格)" props=["AllObjs[]", "Left"]() -> ("AllObjs[]"=w12:refnum<vi>[])  [unwired: 2 in, 3 out]
  n43 = property on="Output" class="Clust (严格)" props=["AllObjs[]", "Left"]() -> ("AllObjs[]"=w11:refnum<vi>[])  [unwired: 2 in, 3 out]
  n44 = while {
    tunnel: w17 -> [w113]
    tunnel: w16 -> [w112]
    tunnel: w14 -> [w111]
    shift-right: [w108] -> _
    shift-left: enum16{"Null", "Operator", "Administrator"}."Null" ("当前用户:") -> [w109]
    shift-right: [w107] -> _
    shift-left: _ -> [w106]
    shift-right: [w105] -> _
    shift-left: _ -> [w104]
    shift-right: [w103] -> _
    shift-left: _ -> [w102]
    shift-right: [w101] -> _
    shift-left: _ -> [w100]
    shift-right: [w99] -> _
    shift-left: _ -> [w98]
    stop <- FALSE stop-if-true
    n45 = event shown="[6] \"用户变更\": 值改变" {
      selector: _ -> [_ _ _ _ _ _ _ _]
      dyn-events: _ -> [_ _ _ _ _ _ _ _]
      timeout: _ -> [_ _ _ _ _ _ _ _]
      tunnel: w113 -> [_ w123 w132 w141 w149 _ _ _]
      tunnel: w112 -> [_ w118 w127 w138 w145 _ _ _]
      tunnel: [_ w121 w130 w136 w144 w151 w185 w192] -> w101
      tunnel: w111 -> [_ w122 w129 w137 _ _ _ _]
      tunnel: [_ w120 w131 w140 w148 w154 w188 w195] -> w107
      tunnel: [_ w119 w128 w139 w147 w153 w187 w194] -> w105
      tunnel: [_ w117 w126 w135 w146 w152 w186 w193] -> w103
      tunnel: [_ enum32{"用户管理", "伺服监控", "产量数据", "状态监控"}."用户管理" ("左侧菜单选项卡") enum32{"用户管理", "伺服监控", "产量数据", "状态监控"}."伺服监控" ("左侧菜单选项卡") enum32{"用户管理", "伺服监控", "产量数据", "状态监控"}."产量数据" ("左侧菜单选项卡") enum32{"用户管理", "伺服监控", "产量数据", "状态监控"}."状态监控" ("左侧菜单选项卡") w150 w184 w191] -> w99
      tunnel: w109 -> [w114 w115 w124 w133 w142 w155 w183 w196]
      tunnel: [w114 w115 w124 w133 w142 w156 w183 w197] -> w108
      tunnel: w106 -> [_ _ _ _ _ w154 w188 w195]
      tunnel: w104 -> [_ _ _ _ _ w153 w187 w194]
      tunnel: w102 -> [_ _ _ _ _ w152 w186 w193]
      tunnel: w100 -> [_ _ _ _ _ w151 w185 w192]
      tunnel: w98 -> [_ _ _ _ _ w150 w184 w191]
      event Timeout {
        n46 = event-data() -> ()  [unwired: 1 in, 1 out]
      }
      event "1": Value Change {
        n47 = event-data() -> ()  [unwired: 1 in, 1 out]
        n48 = Add(x=w123, y=w118) -> (x+y=w121:u32)
        n49 = Add(x=w121, y=w122) -> (x+y=w120:u32)
        n50 = Add(x=w120, y=w118) -> (x+y=w119:u32)
        n51 = Add(x=w119, y=w118) -> (x+y=w117:u32)
      }
      event "2": Value Change {
        n52 = event-data() -> ()  [unwired: 1 in, 1 out]
        n53 = Add(x=w132, y=w127) -> (x+y=w131:u32)
        n54 = Add(x=w131, y=w127) -> (x+y=w130:u32)
        n55 = Add(x=w129, y=w130) -> (x+y=w128:u32)
        n56 = Add(x=w128, y=w127) -> (x+y=w126:u32)
      }
      event "3": Value Change {
        n57 = event-data() -> ()  [unwired: 1 in, 1 out]
        n58 = Add(x=w141, y=w138) -> (x+y=w140:u32)
        n59 = Add(x=w140, y=w138) -> (x+y=w139:u32)
        n60 = Add(x=w139, y=w138) -> (x+y=w136:u32)
        n61 = Add(x=w137, y=w136) -> (x+y=w135:u32)
      }
      event "4": Value Change {
        n62 = event-data() -> ()  [unwired: 1 in, 1 out]
        n63 = Add(x=w149, y=w145) -> (x+y=w148:u32)
        n64 = Add(x=w148, y=w145) -> (x+y=w147:u32)
        n65 = Add(x=w147, y=w145) -> (x+y=w146:u32)
        n66 = Add(x=w146, y=w145) -> (x+y=w144:u32)
      }
      event "确认变更": Value Change {
        n67 = event-data() -> ()  [unwired: 1 in, 1 out]
        n68 = Not Equal?(x="请选择用户:", y=w155) -> (x != y?=w157:bool)
        n69 = case shown="真" w157 {
          tunnel: "请选择用户:" -> [_ w163]
          tunnel: [w159 w165] -> w156
          tunnel: w155 -> [w159 w164]
          frame False {
            n70 = One Button Dialog(message="当前已为该用户!!" ("消息")) -> ()  [unwired: 1 in, 1 out]
          }
          frame True {
            n71 = Equal?(x=w163, y=enum16{"Null", "Operator", "Administrator"}."Operator" ("当前用户:")) -> (x = y?=w170:bool)
            n72 = Equal?(x=w163, y=enum16{"Null", "Operator", "Administrator"}."Administrator" ("当前用户:")) -> (x = y?=w172:bool)
            n73 = Equal?(x="请输入密码:", y="000") -> (x = y?=w171:bool)
            n74 = Equal?(x="请输入密码:", y="123") -> (x = y?=w169:bool)
            n75 = And(x=w172, y=w171) -> (x .and. y?=w168:bool)
            n76 = And(x=w170, y=w169) -> (x .and. y?=w167:bool)
            n77 = Or(x=w168, y=w167) -> (x .or. y?=w166:bool)
            n78 = case shown="真" w166 {
              tunnel: w164 -> [w177 _]
              tunnel: [w177 w178] -> w165
              tunnel: w163 -> [_ w178]
              frame False {
                n79 = One Button Dialog(message="密码错误!!" ("消息")) -> ()  [unwired: 1 in, 1 out]
              }
              frame True {
              }
            }
          }
        }
      }
      event "用户变更": Value Change {
        n80 = event-data() -> ()  [unwired: 1 in, 1 out]
        n81 = case shown="真" "用户变更" {
          tunnel: [w189 w190] -> w182
          tunnel: [w189 w190] -> w181
          tunnel: [w189 w190] -> w180
          frame False {
            w189 = FALSE
          }
          frame True {
            w190 = TRUE
          }
        }
        n82 = property on="确认变更" class="Bool"("Visible"=w180) -> ()  [unwired: 2 in, 2 out]
        n83 = property on="请选择用户:" class="Enum (严格)"("Visible"=w182) -> ()  [unwired: 2 in, 2 out]
        n84 = property on="请输入密码:" class="Str"("Visible"=w181) -> ()  [unwired: 2 in, 2 out]
      }
      event "用户登出": Value Change {
        n85 = event-data() -> ()  [unwired: 1 in, 1 out]
        n86 = Two Button Dialog(message="确认退出吗?" ("消息")) -> (T button?=w198:bool)  [unwired: 2 in]
        n87 = case shown="真" w198 {
          tunnel: [w200 enum16{"Null", "Operator", "Administrator"}."Null" ("当前用户:")] -> w197
          tunnel: w196 -> [w200 _]
          frame False {
          }
          frame True {
          }
        }
      }
    }
    "当前用户:" <- w108
    n88 = property on="3" class="Bool"("Top"=w105) -> ()  [unwired: 2 in, 2 out]
    n89 = property on="4" class="Bool"("Top"=w103) -> ()  [unwired: 2 in, 2 out]
    n90 = property on="2" class="Bool"("Top"=w107) -> ()  [unwired: 2 in, 2 out]
    n91 = property on="左侧菜单选项卡" class="TabCtl (严格)"("Value"=w99) -> ()  [unwired: 2 in, 2 out]
    n92 = property on="左侧菜单选项卡" class="TabCtl (严格)"("Top"=w101) -> ()  [unwired: 2 in, 2 out]
  }
  n93 = call-poly <vilib>:"DB Tools Open Connection.vi"("connection information"="[oledb]\n; Everything after this line is an OLE DB initstring\nProvider=MSDASQL.1;Persist Security Info=False;User ID=root;Data Source=LabviewMysql\n") -> ("error out"=w5:errorcluster, "connection reference"=w9:T12)  [unwired: 7 in]
  n94 = call <vilib>:"DB Tools List Tables.vi"("error in (no error)"=w5, "connection reference"=w9) -> ("error out"=w4:errorcluster, "tables"=w6:string[], "connection reference out"=w8:T12)  [unwired: 3 in]
  n95 = while {
    tunnel: w12 -> [w204]
    tunnel: w11 -> [w202]
    stop <- FALSE stop-if-true
    n96 = for {
      tunnel: w204 -> [w210] mode=indexing
      tunnel: "IO监控滚动条" -> [w209]
      tunnel: w202 -> [w207] mode=indexing
      n97 = Multiply(x=w209, y=-30) -> (x*y=w206:i32)
      n98 = property class="GObj"(reference=w210, "Left"=w206) -> ()  [unwired: 1 in, 2 out]
      n99 = property class="GObj"(reference=w207, "Left"=w206) -> ()  [unwired: 1 in, 2 out]
    }
  }
  n100 = while {
    tunnel: w8 -> [w224]
    tunnel: [w223] -> w7
    tunnel: w6 -> [w222]
    shift-right: [w221] -> _
    shift-left: _ -> [w219]
    shift-right: [w220] -> _
    shift-left: _ -> [w216]
    shift-right: [w217] -> _
    shift-left: _ -> [w218]
    shift-right: [w215] -> _
    shift-left: _ -> [w214]
    shift-right: [w212] -> w3
    shift-left: w4 -> [w213]
    stop <- w211 stop-if-true
    n101 = case shown="无错误" w213 {
      selector: w213 -> [w226 w533]
      tunnel: w224 -> [w237 w534]
      tunnel: [w236 w534] -> w223
      tunnel: w222 -> [w235 _]
      tunnel: [w234 _] -> w221
      tunnel: [w233 _] -> w220
      tunnel: w219 -> [w232 _]
      tunnel: w218 -> [w231 _]
      tunnel: [w230 _] -> w217
      tunnel: w216 -> [w229 _]
      tunnel: [w228 _] -> w215
      tunnel: w214 -> [w227 _]
      tunnel: [w225 w533] -> w212
      tunnel: [_ TRUE] -> w211
      frame No Error {
        n102 = event shown="[3] \"下一页\": 值改变" {
          selector: _ -> [_ _ _ _]
          dyn-events: _ -> [_ _ _ _]
          timeout: _ -> [_ _ _ _]
          tunnel: w237 -> [w259 w300 _ _]
          tunnel: [w255 _ _ _] -> w236
          tunnel: w235 -> [w254 w301 _ _]
          tunnel: [1 1 w500 w516] -> w234
          tunnel: [w245 w263 w496 w515] -> w233
          tunnel: w232 -> [_ _ w502 w517]
          tunnel: [w239 w262 w498 w518] -> w230
          tunnel: w231 -> [_ _ w501 w521]
          tunnel: w229 -> [_ _ w496 w515]
          tunnel: [w244 w268 w499 w520] -> w228
          tunnel: w227 -> [_ _ w497 w519]
          tunnel: w226 -> [w241 w261 _ _]
          tunnel: [w238 w260 _ _] -> w225
          event "刷新": Value Change {
            w242 = timestamp(0 s since 1904-01-01)
            n103 = event-data() -> ()  [unwired: 1 in, 1 out]
            n104 = Index Array(array=w254, index=0 ("索引")) -> (element=w252:string)
            n105 = call <vilib>:"DB Tools List Columns.vi"("error in (no error)"=w241, "table"=w252, "connection reference"=w259) -> ("error out"=w240:errorcluster, "columns"=w256:string[], "connection reference out"=w258:T12)  [unwired: 1 in, 1 out]
            n106 = property on="数据查询" class="Tbl (严格)"("Column Headers[]"=w256) -> ()  [unwired: 2 in, 2 out]
            n107 = call <vilib>:"DB Tools Select All Data.vi"("error in (no error)"=w240, "table"=w252, "connection reference"=w258) -> ("error out"=w238:errorcluster, "data"=w239:string[][], "connection reference out"=w255:T12)  [unwired: 3 in]
            n108 = Array Subset(array=w239, length (row)=20 ("长度")) -> (w244:string[][])  [unwired: 3 in]
            n109 = property on="关键字查询" class="Str"("Value"="") -> ()  [unwired: 2 in, 2 out]
            n110 = property on="终结时间" class="AbsTime (严格)"("Value"=w242) -> ()  [unwired: 2 in, 2 out]
            n111 = property on="起始时间" class="AbsTime (严格)"("Value"=w242) -> ()  [unwired: 2 in, 2 out]
            n112 = Array Size(array=w239) -> (size(s)=w250:i32[])
            n113 = Index Array(array=w250, index=0 ("索引")) -> (element=w248:i32)
            n114 = Divide(x=w248, y=20) -> (x/y=w246:dbl)
            n115 = Round Toward +Infinity(x=w246) -> (ceil(x): smallest int >= x=w245:dbl)
          }
          event "查询": Value Change {
            w297 = timestamp(0 s since 1904-01-01)
            n116 = event-data() -> ()  [unwired: 1 in, 1 out]
            n117 = Index Array(array=w301, index=0 ("索引")) -> (element=w299:string)
            n118 = Not Equal?(x="关键字查询", y="") -> (x != y?=w296:bool)
            n119 = Not Equal?(x="终结时间", y=w297) -> (x != y?=w295:bool)
            n120 = Not Equal?(x="起始时间", y=w297) -> (x != y?=w294:bool)
            n121 = case shown="真" w296 {
              tunnel: w295 -> [w306 w402]
              tunnel: w294 -> [w307 w401]
              tunnel: "where " -> [w308 w400]
              tunnel: " intro " -> [_ w398]
              tunnel: [w320 w399] -> w290
              tunnel: [w319 w397] -> w289
              tunnel: [w318 w396] -> w288
              tunnel: [w317 w395] -> w287
              tunnel: "关键字查询" -> [_ w394]
              tunnel: [w316 w393] -> w286
              tunnel: [w315 w392] -> w285
              tunnel: [w314 w391] -> w284
              tunnel: " signTime " -> [w305 w390]
              tunnel: "起始时间" -> [w303 w389]
              tunnel: "终结时间" -> [w304 w388]
              tunnel: [w313 w387] -> w279
              tunnel: [w312 w386] -> w280
              tunnel: [w311 w385] -> w277
              tunnel: [w310 w384] -> w278
              tunnel: [w309 w383] -> w276
              tunnel: [_ w382] -> w275
              tunnel: [_ w381] -> w274
              frame False {
                n122 = case shown="假" w307 {
                  tunnel: [w336 w356] -> w320
                  tunnel: [w335 w354] -> w319
                  tunnel: [w334 w352] -> w318
                  tunnel: [w333 w351] -> w317
                  tunnel: [w332 w350] -> w316
                  tunnel: [w331 w348] -> w315
                  tunnel: [w330 w347] -> w314
                  tunnel: [w329 w345] -> w313
                  tunnel: [w328 _] -> w312
                  tunnel: [w327 _] -> w311
                  tunnel: [w326 _] -> w310
                  tunnel: [w325 _] -> w309
                  tunnel: w308 -> [w324 w357]
                  tunnel: w306 -> [w323 w355]
                  tunnel: w305 -> [w322 w353]
                  tunnel: w304 -> [w321 w346]
                  tunnel: w303 -> [_ w349]
                  frame False {
                    n123 = case shown="假" w323 {
                      tunnel: [w337 w344] -> w336
                      tunnel: [w337 w343] -> w335
                      tunnel: [w337 " <= "] -> w334
                      tunnel: [w337 w338] -> w333
                      tunnel: [w337 _] -> w332
                      tunnel: [w337 _] -> w331
                      tunnel: [w337 _] -> w330
                      tunnel: [w337 _] -> w329
                      tunnel: [w337 _] -> w328
                      tunnel: [w337 _] -> w327
                      tunnel: [w337 _] -> w326
                      tunnel: [w337 _] -> w325
                      tunnel: w324 -> [_ w344]
                      tunnel: w322 -> [_ w343]
                      tunnel: w321 -> [_ w341]
                      frame False {
                        w337 = ""
                      }
                      frame True {
                        w339 = "'"
                        n124 = Format Date/Time String(seconds (now)=w341) -> (date/time string=w340:string)  [unwired: 2 in]
                        n125 = Concatenate Strings(w339, w340, w339) -> (w338:string)
                      }
                    }
                  }
                  frame True {
                    n126 = case shown="假" w355 {
                      tunnel: w357 -> [w364 w377]
                      tunnel: [w364 w377] -> w356
                      tunnel: [w363 w370] -> w354
                      tunnel: w353 -> [w363 w370]
                      tunnel: [" >= " " >= "] -> w352
                      tunnel: [w358 w372] -> w351
                      tunnel: [_ " and "] -> w350
                      tunnel: w349 -> [w361 w375]
                      tunnel: [_ w370] -> w348
                      tunnel: [_ " <= "] -> w347
                      tunnel: w346 -> [_ w368]
                      tunnel: [_ w365] -> w345
                      frame False {
                        w359 = "'"
                        n127 = Format Date/Time String(seconds (now)=w361) -> (date/time string=w360:string)  [unwired: 2 in]
                        n128 = Concatenate Strings(w359, w360, w359) -> (w358:string)
                      }
                      frame True {
                        w366 = "'"
                        w373 = "'"
                        n129 = Format Date/Time String(seconds (now)=w375) -> (date/time string=w374:string)  [unwired: 2 in]
                        n130 = Format Date/Time String(seconds (now)=w368) -> (date/time string=w367:string)  [unwired: 2 in]
                        n131 = Concatenate Strings(w366, w367, w366) -> (w365:string)
                        n132 = Concatenate Strings(w373, w374, w373) -> (w372:string)
                      }
                    }
                  }
                }
              }
              frame True {
                n133 = case shown="真" w401 {
                  tunnel: w402 -> [w411 w465]
                  tunnel: w400 -> [w421 w464]
                  tunnel: [w420 w463] -> w399
                  tunnel: w398 -> [w419 w462]
                  tunnel: [w418 w461] -> w397
                  tunnel: [w416 w460] -> w396
                  tunnel: [w414 w459] -> w395
                  tunnel: w394 -> [w413 w458]
                  tunnel: [w412 w457] -> w393
                  tunnel: [w409 w456] -> w392
                  tunnel: [w408 w455] -> w391
                  tunnel: w390 -> [w407 w454]
                  tunnel: w389 -> [_ w453]
                  tunnel: w388 -> [w404 w452]
                  tunnel: [w406 w451] -> w387
                  tunnel: [w405 w450] -> w386
                  tunnel: [_ w449] -> w385
                  tunnel: [w403 w448] -> w384
                  tunnel: [_ w447] -> w383
                  tunnel: [_ w446] -> w382
                  tunnel: [_ w445] -> w381
                  tunnel: "like " -> [w417 w444]
                  tunnel: " '%" -> [w415 w443]
                  tunnel: "%' " -> [w410 w442]
                  frame False {
                    n134 = case shown="真" w411 {
                      tunnel: w421 -> [w427 w440]
                      tunnel: [w427 w440] -> w420
                      tunnel: w419 -> [w426 w439]
                      tunnel: [w426 w439] -> w418
                      tunnel: [w425 w438] -> w416
                      tunnel: w417 -> [w425 w438]
                      tunnel: [w424 w437] -> w414
                      tunnel: w415 -> [w424 w437]
                      tunnel: w413 -> [w423 w436]
                      tunnel: [w423 w436] -> w412
                      tunnel: [w422 w435] -> w409
                      tunnel: w410 -> [w422 w435]
                      tunnel: [_ "and"] -> w408
                      tunnel: w407 -> [_ w433]
                      tunnel: [_ w433] -> w406
                      tunnel: [_ " <= "] -> w405
                      tunnel: w404 -> [_ w431]
                      tunnel: [_ w428] -> w403
                      frame False {
                      }
                      frame True {
                        w429 = "'"
                        n135 = Format Date/Time String(seconds (now)=w431) -> (date/time string=w430:string)  [unwired: 2 in]
                        n136 = Concatenate Strings(w429, w430, w429) -> (w428:string)
                      }
                    }
                  }
                  frame True {
                    n137 = case shown="真" w465 {
                      tunnel: w464 -> [w478 w495]
                      tunnel: [w478 w495] -> w463
                      tunnel: w462 -> [w477 w494]
                      tunnel: [w477 w494] -> w461
                      tunnel: [w476 w482] -> w460
                      tunnel: [w475 w481] -> w459
                      tunnel: w458 -> [w474 w493]
                      tunnel: [w474 w493] -> w457
                      tunnel: [w473 w480] -> w456
                      tunnel: [w472 w479] -> w455
                      tunnel: w454 -> [w471 w487]
                      tunnel: w453 -> [w467 w491]
                      tunnel: w452 -> [_ w490]
                      tunnel: [w471 w487] -> w451
                      tunnel: [" >= " " >= "] -> w450
                      tunnel: [_ w479] -> w449
                      tunnel: [w466 w488] -> w448
                      tunnel: [_ w487] -> w447
                      tunnel: [_ " ;= "] -> w446
                      tunnel: [_ w483] -> w445
                      tunnel: w444 -> [w476 w482]
                      tunnel: w443 -> [w475 w481]
                      tunnel: w442 -> [w473 w480]
                      tunnel: " and " -> [w472 w479]
                      frame False {
                        w468 = "'" ("字符串")
                        n138 = Format Date/Time String(seconds (now)=w467) -> (date/time string=w469:string)  [unwired: 2 in]
                        n139 = Concatenate Strings(w468, w469, w468) -> (w466:string)
                      }
                      frame True {
                        w484 = "'"
                        n140 = Format Date/Time String(seconds (now)=w491) -> (date/time string=w489:string)  [unwired: 2 in]
                        n141 = Format Date/Time String(seconds (now)=w490) -> (date/time string=w485:string)  [unwired: 2 in]
                        n142 = Concatenate Strings(w484, w489, w484) -> (w488:string)
                        n143 = Concatenate Strings(w484, w485, w484) -> (w483:string)
                      }
                    }
                  }
                }
              }
            }
            n144 = Concatenate Strings(w290, w289, w288, w287, w286, w285, w284, w279, w280, w278, w277, w276, w275, w274) -> (w273:string)
            "连接的字符串" <- w273
            n145 = call <vilib>:"DB Tools Select Data.vi"("condition"=w273, "error in (no error)"=w261, "table"=w299, "connection reference"=w300) -> ("error out"=w260:errorcluster, "data"=w272:variant[][])  [unwired: 2 in, 1 out]
            n146 = Variant To Data(type=string[][] [], Variant=w272) -> (data=w262:string[][])  [unwired: 1 in, 1 out]
            n147 = Array Subset(array=w262, length (row)=20 ("长度")) -> (w268:string[][])  [unwired: 3 in]
            n148 = Array Size(array=w262) -> (size(s)=w267:i32[])
            n149 = Index Array(array=w267) -> (element=w265:i32)  [unwired: 1 in]
            n150 = Divide(x=w265, y=20) -> (x/y=w266:dbl)
            n151 = Round Toward +Infinity(x=w266) -> (ceil(x): smallest int >= x=w263:dbl)
          }
          event "上一页": Value Change {
            n152 = event-data() -> ()  [unwired: 1 in, 1 out]
            n153 = Less?(x=1, y=w502) -> (x < y?=w503:bool)
            n154 = case shown="真" w503 {
              tunnel: w502 -> [w507 w514]
              tunnel: w501 -> [w506 w510]
              tunnel: [w505 w513] -> w499
              tunnel: [w507 w509] -> w500
              tunnel: [w506 w510] -> w498
              tunnel: w497 -> [w505 _]
              frame False {
              }
              frame True {
                w511 = 20 ("x")
                n155 = Decrement(x=w514) -> (x-1=w509:i32)
                n156 = Decrement(x=w509) -> (x-1=w508:i32)
                n157 = Multiply(x=w511, y=w508) -> (x*y=w512:i32)
                n158 = Array Subset(array=w510, index (row)=w512, length (row)=w511) -> (w513:string[][])  [unwired: 2 in]
              }
            }
          }
          event "下一页": Value Change {
            n159 = event-data() -> ()  [unwired: 1 in, 1 out]
            n160 = Less?(x=w517, y=w515) -> (x < y?=w522:bool)
            n161 = case shown="真" w522 {
              tunnel: w521 -> [w524 w530]
              tunnel: [w525 w531] -> w520
              tunnel: w519 -> [w525 _]
              tunnel: [w524 w530] -> w518
              tunnel: w517 -> [w523 w526]
              tunnel: [w523 w529] -> w516
              frame False {
              }
              frame True {
                w527 = 20 ("x")
                n162 = Increment(x=w526) -> (x+1=w529:i32)
                n163 = Multiply(x=w527, y=w526) -> (x*y=w528:i32)
                n164 = Array Subset(array=w530, index (row)=w528, length (row)=w527) -> (w531:string[][])  [unwired: 2 in]
              }
            }
          }
        }
      }
      frame Error {
      }
    }
    "当前页数" <- w221
    "总页数" <- w220
    "data" <- w217
    "数据查询" <- w215
  }
  n165 = call <vilib>:"DB Tools Close Connection.vi"("error in (no error)"=w3, "connection reference"=w7) -> ("error out"=w2:errorcluster)  [unwired: 5 in]
  n166 = call <vilib>:"Simple Error Handler.vi"("error in (no error)"=w2) -> ("error out"=→"error out":errorcluster)  [unwired: 4 in, 4 out]
